vi "fpga_test_cavity.vi"() -> ()   [LabVIEW 2013]
uses:
  <vilib>/Platform/TimedLoop/XDataNode/timing_clust.ctl
  <vilib>/Platform/TimedLoop/XDataNode/nitl_modes.ctl
  <vilib>/Platform/TimedLoop/XDataNode/wakeup.ctl
  <vilib>/rvi/Emulation/niFpgaSctlEmulationGetInTimedLoop.vi
  <vilib>/rvi/Emulation/niFpgaEmulationReportErrorSimple.vi
  <vilib>/rvi/Emulation/niFpgaGetClockAttributes.vi
  <vilib>/rvi/Emulation/niFpgaCriticalErrorInLSC.vi
  <vilib>/rvi/interface/RandomDataEmulation/nirviRandomDataMultiElementFPGAFIFO.vi
  <instcachedir>/0/nirviRandomDataMultiElementFPGAFIFO_F2B80EDE0D7944A08478D8D26097D4DB.lvgen/nirviRandomDataMultiElementFPGAFIFO_F2B80EDE0D7944A08478D8D26097D4DB_005.vi
  <vilib>/rvi/interface/RandomDataEmulation/niFpgaRandomDataHandleErrors.vi
  <vilib>/Platform/TimedLoop/XDataNode/XDataNode.xnode
  <vilib>/rvi/FXPMathLib/FxpInterpret/XNode/nifxpmath_Interpret.xnode
  <vilib>/rvi/DataTransferAndStorage/Container/XNode/niFpgaContainer.xnode
  <vilib>/rvi/interface/RandomDataEmulation/nirviRandomDataFpgaMultiElementTemplate.vi
  <vilib>/Platform/TimedLoop/XDataNode/XDNodeRunTimeDep.lvlib
panel:
  in  "Start":bool
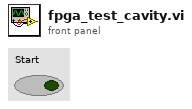
[diagram p1: front panel]
types:
  T1 = typedef "XDNodeRunTimeDep.lvlib/timing_clust.ctl" = cluster{"Expected End [f-1]":u64, "Actual End [f-1]":u64, "Finished Late? [f-1]":bool, "Expected End [i-1]":u64, "Actual End [i-1]":u64, "Finished Late? [i-1]":bool, "Expected Start [i]":u64, "Actual Start [i]":u64, "Expected Start [f]":u64, "Actual Start [f]":u64, "Source Name":string, "Structure Name":string, "Period":i64, "Deadline":i64, "Offset":i64, "Start":i64, "Priority":i32, "Timeout":i32, "Mode":T2, "Wakeup Reason":T3, "Error":errorcluster, "Source Type":string, "Secondary Source Type":string, "Global End Time":u64, "Global Start Time":u64, "Frame Duration":u64, "Iteration Duration":u64, "Assigned CPU":i32, "I/O Scan Engine Mode":u32}
  T2 = typedef "XDNodeRunTimeDep.lvlib/nitl_modes.ctl" = enum32{"No Change", "Process missed periods, maintain original phase", "Discard missed periods, maintain original phase", "Process missed periods, ignore original phase", "Discard missed periods, ignore original phase"}
  T3 = typedef "XDNodeRunTimeDep.lvlib/wakeup.ctl" = enum32{"Normal", "Aborted", "Asynchronous wakeup", "Timing source error", "Timed loop error", "Timeout"}
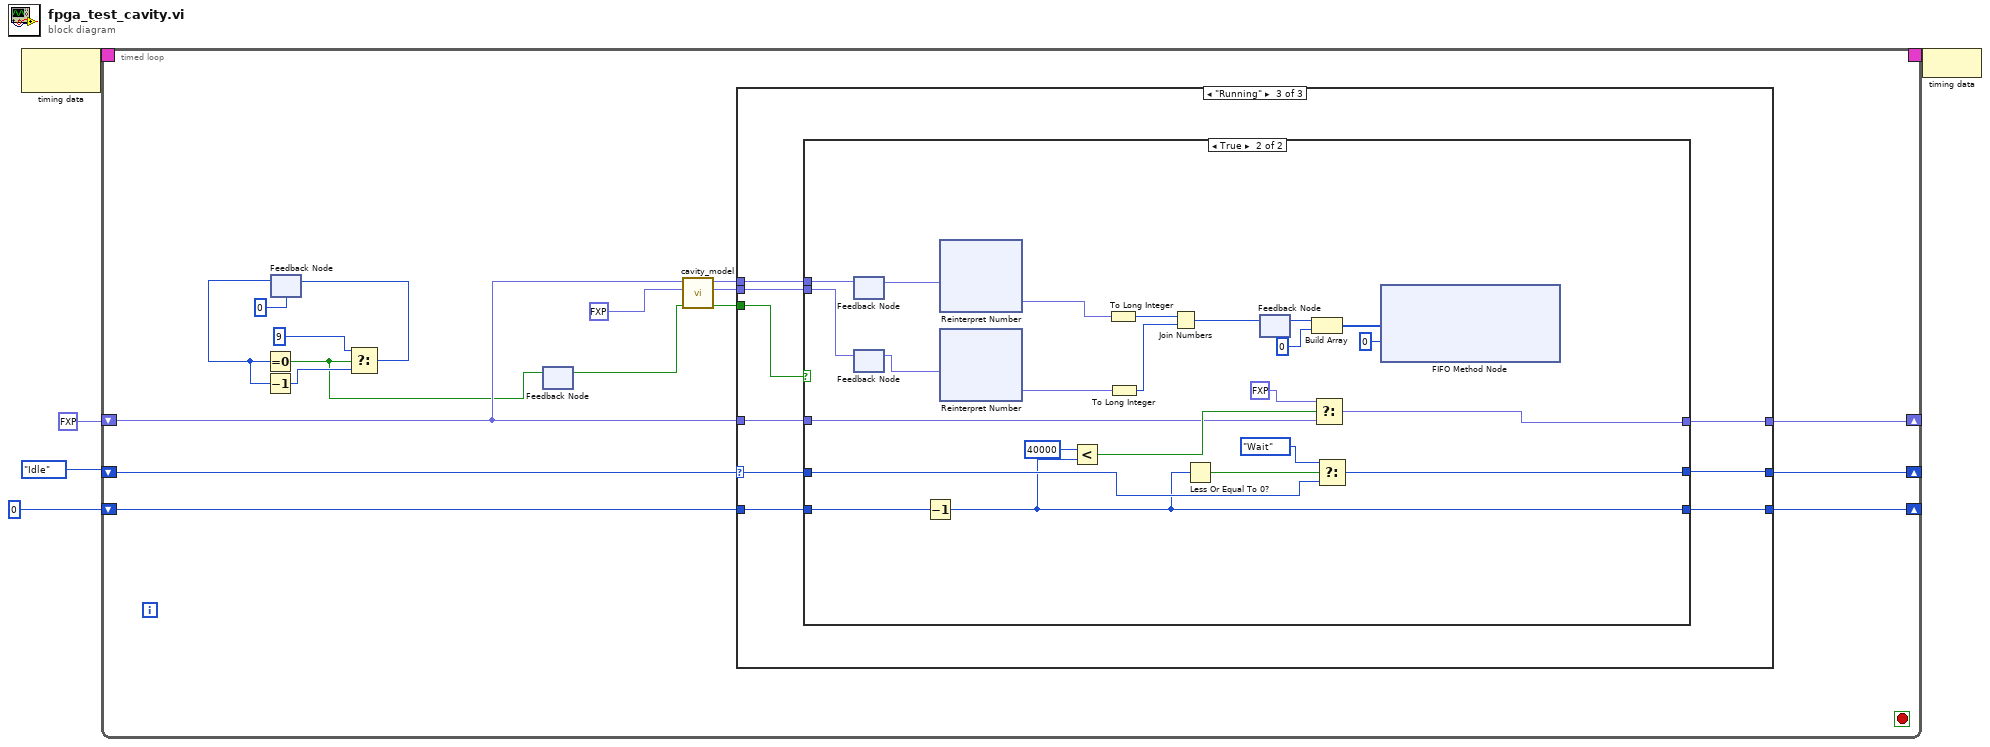
[diagram p0: block diagram]
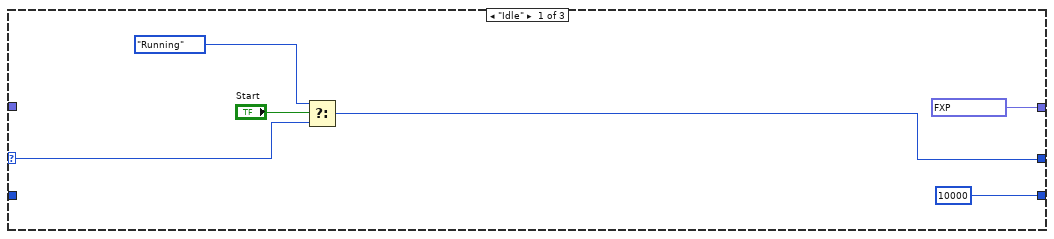
[diagram p2: hidden frame]
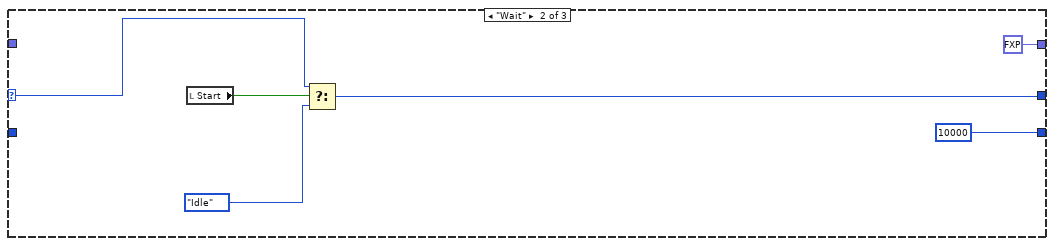
[diagram p3: hidden frame]
diagram:
  n1 = node-c288() -> (w5:T1)  [unwired: 1 in]
  n2 = timed-loop {
    timing: w5 -> [_]
    timing-out: [_] -> w4
    shift-right: [w18] -> _
    shift-left: enum16{"Idle", "Running", "Wait"}."Idle" -> [w19]
    shift-right: [w17] -> _
    shift-left: u16 0 -> [w15]
    shift-right: [w14] -> _
    shift-left: fxp<+/-,16,1> 0.0 ("Ii") -> [w13]
    stop <- _ stop-if-true
    n3 = feedback #1(i8 0) -> (w11:i8)
    n4 = Equal To 0?(x=w11) -> (x = 0?=w7:bool)
    n5 = Decrement(x=w11) -> (x-1=w10:i8)
    n6 = Select(t=i8 9, s=w7, f=w10) -> (s? t:f=w8:i8)
    n7 = feedback-in #1(w8) -> ()
    n8 = feedback-in #2(w7) -> ()
    n9 = feedback #2() -> (w6:bool)  [unwired: 1 in]
    n10 = call "cavity_model.vi"("input valid"=w6, "Ii"=fxp<+/-,16,1> 0.0, "Ir"=w13) -> ("output valid"=w16:bool, "Vi"=w20:fxp<+/-,32,26>, "Vr"=w21:fxp<+/-,32,26>)  [unwired: 6 in]
    n11 = case shown="\"Running\"" w19 {
      selector: w19 -> [w27 w30 w38]
      tunnel: w21 -> [_ _ w43]
      tunnel: w20 -> [_ _ w42]
      tunnel: [w25 w34 w37] -> w18
      tunnel: [u16 10000 u16 10000 w39] -> w17
      tunnel: w16 -> [_ _ w41]
      tunnel: w15 -> [_ _ w40]
      tunnel: [fxp<+/-,16,1> 0.0029296875 ("Ii") fxp<+/-,16,1> 0.0 ("Ii") w36] -> w14
      tunnel: w13 -> [_ _ w35]
      frame "Idle" {
        n12 = Select(t=enum16{"Idle", "Running", "Wait"}."Running", s="Start", f=w27) -> (s? t:f=w25:enum16{"Idle", "Running", "Wait"})
      }
      frame "Wait" {
        n13 = local read "Start"() -> (w32:bool)
        n14 = Select(t=w30, s=w32, f=enum16{"Idle", "Running", "Wait"}."Idle" ("t")) -> (s? t:f=w34:enum16{"Idle", "Running", "Wait"})
      }
      frame "Running" {
        n15 = case shown="True" w41 {
          tunnel: w43 -> [_ w66]
          tunnel: w42 -> [_ w65]
          tunnel: w40 -> [w45 w58]
          tunnel: [w45 w52] -> w39
          tunnel: w38 -> [w46 w56]
          tunnel: [w46 w55] -> w37
          tunnel: [w44 w48] -> w36
          tunnel: w35 -> [w44 w47]
          frame False {
          }
          frame True {
            n16 = feedback #3() -> (w70:fxp<+/-,32,26>)  [unwired: 1 in]
            n17 = feedback-in #3(w66) -> ()
            n18 = feedback #4() -> (w69:fxp<+/-,32,26>)  [unwired: 1 in]
            n19 = feedback-in #4(w65) -> ()
            n20 = Decrement(x=w58) -> (x-1=w52:u16)
            n21 = xnode "Reinterpret Number"("x"=w70) -> ("y"=w68:fxp<+/-,32,32>)
            n22 = xnode "Reinterpret Number"("x"=w69) -> ("y"=w67:fxp<+/-,32,32>)
            n23 = Less?(x=u16 40000, y=w52) -> (x < y?=w50:bool)
            n24 = To Long Integer(number=w68) -> (32bit integer=w64:i32)
            n25 = To Long Integer(number=w67) -> (32bit integer=w63:i32)
            n26 = Join Numbers(hi=w64, lo=w63) -> ((hi.lo)=w62:u64)
            n27 = Less Or Equal To 0?(x=w52) -> (x <= 0?=w57:bool)
            n28 = feedback #5() -> (w61:u64)  [unwired: 1 in]
            n29 = feedback-in #5(w62) -> ()
            n30 = Build Array(w61, u64 0 ("element")) -> (w60:u64[])
            n31 = Select(t=fxp<+/-,16,1> 0.0 ("Ii"), s=w50, f=w47) -> (s? t:f=w48:fxp<+/-,16,1>)
            n32 = Select(t=enum16{"Idle", "Running", "Wait"}."Wait", s=w57, f=w56) -> (s? t:f=w55:enum16{"Idle", "Running", "Wait"})
            n33 = xnode ("FIFO Method Node")("Element"=w60, "Timeout"=0) -> ()  [unwired: 1 in, 2 out]
          }
        }
      }
    }
  }
  n34 = node-c288(w4) -> ()
